vi "Reset Math Channel.vi"(8 "error in (no error)":errorcluster, 9 "Channel (0: All)":u16(ring) items=["All", "Function 1", "Function 2", "Function 3", "Function 4"], 11 "VISA resource name":refnum<visa-resource-name>) -> (0 "error out":errorcluster, 3 "VISA resource name out":refnum<visa-resource-name>)   [LabVIEW 2015, in "LeCroy Wave Series.lvlib"]
doc: "Resets a waveform processing function."
uses:
  <instrlib>/LeCroy Wave Series/LeCroy Wave Series.lvlib
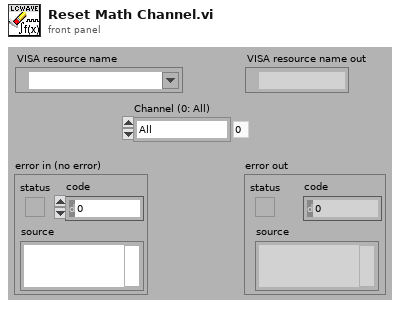
[diagram p1: front panel]
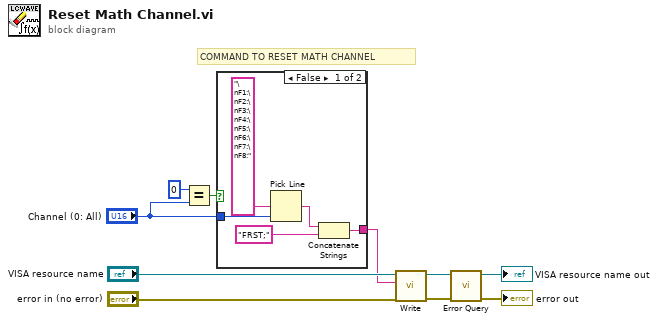
[diagram p0: block diagram]
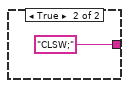
[diagram p2: hidden frame]
diagram:
  # "COMMAND TO RESET MATH CHANNEL"
  n1 = Equal?(x=u16 0, y="Channel (0: All)") -> (x = y?=w7:bool)
  n2 = case shown="False" w7 {
    tunnel: [w11 "CLSW;"] -> w6
    tunnel: "Channel (0: All)" -> [w12 _]
    frame False {
      n3 = Pick Line(multi-line string="\nF1:\nF2:\nF3:\nF4:\nF5:\nF6:\nF7:\nF8:", line index=w12) -> (output string=w14:string)  [unwired: 1 in]
      n4 = Concatenate Strings(w14, "FRST;" ("string")) -> (w11:string)
    }
    frame True {
    }
  }
  n5 = call <instrlib>:"Write.vi"("error in (no error)"="error in (no error)", "Write Buffer"=w6, "VISA resource name"="VISA resource name") -> ("error out"=w3:errorcluster, "VISA resource name out"=w4:refnum<visa-resource-name>)  [unwired: 6 in, 1 out]
  n6 = call <instrlib>:"Error Query.vi"("error in (no error)"=w3, "VISA resource name"=w4) -> ("error out"=→"error out":errorcluster, "VISA resource name out"=→"VISA resource name out":refnum<visa-resource-name>)  [unwired: 6 in, 2 out]
